vi "Query Dwell Time.vi"(8 "error in (no error)":errorcluster, 11 "VISA resource name":refnum<visa-resource-name>) -> (0 "error out":errorcluster, 2 "output":dbl[unit] format="%4_4g", 3 "VISA resource name out":refnum<visa-resource-name>)   [LabVIEW 2015, in "SR400.lvlib"]
doc: "DT { x }\nThe DT command reads and sets the dwell time. If\nx is absent, the dwell time is returned. If x is\nincluded, the dwell time is set to x seconds where\n2E-3 <= x <= 6E1. If x = 0, the dwell is set to\nEXTERNAL. Only the most significant digit of x\nis used so \"DT 2E-3\" , \"DT .0022\" , \"DT 2.2E-3\"\nall set the dwell to 2 ms."
uses:
  SR400.lvlib
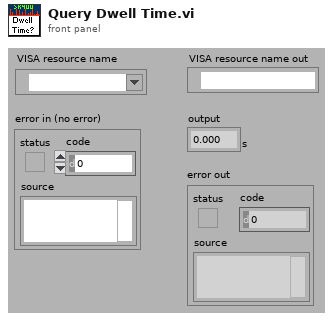
[diagram p1: front panel]
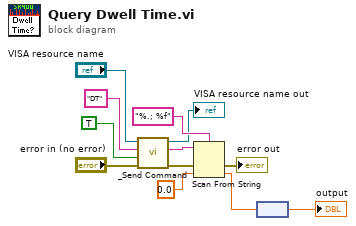
[diagram p0: block diagram]
diagram:
  n1 = call "_Send Command.vi"("error in (no error)"="error in (no error)", "Query? (F)"=TRUE, "Command"="DT" ("command"), "VISA resource name"="VISA resource name") -> ("error out"=w4:errorcluster, "Response"=w5:string, "VISA resource name out"=→"VISA resource name out":refnum<visa-resource-name>)  [unwired: 5 out]
  n2 = Scan From String(format string="%.; %f", input string=w5, error in=w4, default 1=0.0 ("default value 1")) -> (error out=→"error out":errorcluster, output 1=w2:dbl)  [unwired: 1 in, 2 out]
  n3 = node(w2) -> (→"output":dbl[unit])
